vi "ReadConfigFile.vi"(8 "ErrorIn":errorcluster, 11 "ClusterIn":T1={"Admin"={"Lvl"=enum."Admin", "Pwd"=""}, "RTConfig"={"Arm"=FALSE, "Number"=0.0, "String"=""}, "SMS"={"Enbl?"=FALSE, "Addr"=[]}, "FPGA"={"Target"=enum."4", "Channel"=enum."4", "Ref1"=refnum, "Ref2"=refnum}, "Config"={"UsrCfg"={"Paths"={"CfgFile"=path "", "LogFolder"=path "", "LogFile"=path "", "NAS path"=path "", "ThreshFile"=path "", "RedunFolder"=path ""}, "SampleRate"=12500.0}, "FP_User"={"#NoiseSums"=1, "Max_df"=1, "AvgAvg"=FALSE, "#Avg"=1, "AutoCenter"=FALSE, "Inclin"={"Vmin"=0.0, "Vmax"=0.0, "Angle_min"=0.0, "Angle_max"=0.0, "Offset"=0.0, "Pos_Neg"=FALSE}, "1"={"Cal_"={"Fine"=0.999969482421875, "Coarse_"=10000.0}, "Beac"={"Fine"=4194303.0, "Coarse_"=1.0}, "Scale"={"Step4"=10000.0, "Step5"=4194303.0, "Step6"=1.0, "Step7"=10000.0}, "Offset"=1.0, "Scale_Noise"=12500.0, "Scale_Step1"=65535.0, "Scale_In_RT"=1.0, "ScaleMeas"=0.999969482421875, "FreqsToRemove"=[0, 1633], "Width"=[0, 1633], "ScaleMeasEnum"=enum."50", "FilterEnab"=enum."Step 1"}, "2"={"Cal_"={"Fine"=0.000213623046875, "Coarse_"=4194303.0}, "Beac"={"Fine"=0.000213623046875, "Coarse_"=4194303.0}, "Scale"={"Step4"=0.0, "Step5"=4194303.0, "Step6"=1.0, "Step7"=10000.0}, "Offset"=0.0, "Scale_Noise"=4194303.0, "Scale_Step1"=65535.0, "Scale_In_RT"=1.0, "ScaleMeas"=0.999969482421875, "FreqsToRemove"=[0, 1633], "Width"=[0, 1633], "ScaleMeasEnum"=enum."50", "FilterEnab"=enum."Step 1"}, "3"={"Cal_"={"Fine"=0.000213623046875, "Coarse_"=4194303.0}, "Beac"={"Fine"=0.000213623046875, "Coarse_"=4194303.0}, "Scale"={"Step4"=0.0, "Step5"=4194303.0, "Step6"=1.0, "Step7"=10000.0}, "Offset"=0.0, "Scale_Noise"=4194303.0, "Scale_Step1"=65535.0, "Scale_In_RT"=1.0, "ScaleMeas"=0.999969482421875, "FreqsToRemove"=[0, 1633], "Width"=[0, 1633], "ScaleMeasEnum"=enum."50", "FilterEnab"=enum."Step 1"}, "4"={"Cal_"={"Fine"=0.000213623046875, "Coarse_"=4194303.0}, "Beac"={"Fine"=0.000213623046875, "Coarse_"=4194303.0}, "Scale"={"Step4"=0.0, "Step5"=4194303.0, "Step6"=1.0, "Step7"=10000.0}, "Offset"=0.0, "Scale_Noise"=4194303.0, "Scale_Step1"=1.0, "Scale_In_RT"=10000.0, "ScaleMeas"=0.999969482421875, "FreqsToRemove"=[0, 1633], "Width"=[0, 1633], "ScaleMeasEnum"=enum."50", "FilterEnab"=enum."Step 1"}, "Target to Probe"=enum."4", "SNR_Thresh"=1.0, "Paths"={"CfgFile"=path "", "LogFolder"=path "", "LogFile"=path "", "NAS path"=path "", "ThreshFile"=path "", "RedunFolder"=path ""}, "Connex_Location"="", "SimulateFPGA"=FALSE, "Deadband"=0.0}}, "Stat"={"SysState"=enum."Init", "TrackRate"=FALSE, "AutoCentr"=FALSE}, "Alarm"={"TC13"={"Enbl"=FALSE, "ErrsAndWarns"={0.0, 5.663716814159292, 7.168141592920354, 8.584070796460177}}, "AI1"={"Enbl"=FALSE, "ErrsAndWarns"={0.0, 5.663716814159292, 7.168141592920354, 8.584070796460177}}, "AI2"={"Enbl"=FALSE, "ErrsAndWarns"={0.0, 5.663716814159292, 7.168141592920354, 8.584070796460177}}, "AI3"={"Enbl"=FALSE, "ErrsAndWarns"={0.0, 5.663716814159292, 7.168141592920354, 8.584070796460177}}, "AI4"={"Enbl"=FALSE, "ErrsAndWarns"={0.0, 5.663716814159292, 7.168141592920354, 8.584070796460177}}, "AI5"={"Enbl"=FALSE, "ErrsAndWarns"={0.0, 5.663716814159292, 7.168141592920354, 8.584070796460177}}, "AI6"={"Enbl"=FALSE, "ErrsAndWarns"={0.0, 5.663716814159292, 7.168141592920354, 8.584070796460177}}, "AI18"={"Enbl"=FALSE, "ErrsAndWarns"={0.0, 5.663716814159292, 7.168141592920354, 8.584070796460177}}, "AI19"={"Enbl"=FALSE, "ErrsAndWarns"={0.0, 5.663716814159292, 7.168141592920354, 8.584070796460177}}, "TE1"={"Enbl"=FALSE, "ErrsAndWarns"={0.0, 5.663716814159292, 7.168141592920354, 8.584070796460177}}, "TE2"={"Enbl"=TRUE, "ErrsAndWarns"={0.0, 5.663716814159292, 7.168141592920354, 8.584070796460177}}, "TE3"={"Enbl"=FALSE, "ErrsAndWarns"={0.0, 5.663716814159292, 7.168141592920354, 8.584070796460177}}, "ADAM1"={"Enbl"=FALSE, "ErrsAndWarns"={0.0, 5.663716814159292, 7.168141592920354, 8.584070796460177}}, "ADAM2"={"Enbl"=FALSE, "ErrsAndWarns"={0.0, 5.663716814159292, 7.168141592920354, 8.584070796460177}}, "ADAM3"={"Enbl"=FALSE, "ErrsAndWarns"={0.0, 5.663716814159292, 7.168141592920354, 8.584070796460177}}, "ADAM4"={"Enbl"=FALSE, "ErrsAndWarns"={0.0, 5.663716814159292, 7.168141592920354, 8.584070796460177}}, "72CoBeacFreq"={"Enbl"=FALSE, "ErrsAndWarns"={0.0, 5.663716814159292, 7.168141592920354, 8.584070796460177}}, "72CoCalFreq"={"Enbl"=FALSE, "ErrsAndWarns"={0.0, 5.663716814159292, 7.168141592920354, 8.584070796460177}}, "84CoBeacFreq"={"Enbl"=FALSE, "ErrsAndWarns"={0.0, 5.663716814159292, 7.168141592920354, 8.584070796460177}}, "84CoCalFreq"={"Enbl"=FALSE, "ErrsAndWarns"={0.0, 5.663716814159292, 7.168141592920354, 8.584070796460177}}, "72Co_CalTonePwr"={"Enbl"=FALSE, "ErrsAndWarns"={0.0, 5.663716814159292, 7.168141592920354, 8.584070796460177}}, "72X_CalTonePwr"={"Enbl"=FALSE, "ErrsAndWarns"={0.0, 5.663716814159292, 7.168141592920354, 8.584070796460177}}, "84Co_CalTonePwr"={"Enbl"=FALSE, "ErrsAndWarns"={0.0, 5.663716814159292, 7.168141592920354, 8.584070796460177}}, "84X_CalTonePwr"={"Enbl"=FALSE, "ErrsAndWarns"={0.0, 5.663716814159292, 7.168141592920354, 8.584070796460177}}}} {"Alarm"."84X_CalTonePwr"."ErrsAndWarns" scale=-120.0..-45.0; "Alarm"."72X_CalTonePwr"."ErrsAndWarns" scale=-120.0..-45.0; "Alarm"."84Co_CalTonePwr"."ErrsAndWarns" scale=-120.0..-45.0; "Alarm"."72Co_CalTonePwr"."ErrsAndWarns" scale=-120.0..-45.0; "Alarm"."84CoCalFreq"."ErrsAndWarns" scale=24.9..25.1; "Alarm"."84CoBeacFreq"."ErrsAndWarns" scale=25.5..27.0; "Alarm"."72CoCalFreq"."ErrsAndWarns" scale=24.9..25.1; "Alarm"."72CoBeacFreq"."ErrsAndWarns" scale=25.5..27.0; "Alarm"."ADAM4"."ErrsAndWarns" scale=30.0..52.0; "Alarm"."ADAM3"."ErrsAndWarns" scale=30.0..52.0; "Alarm"."ADAM2"."ErrsAndWarns" scale=30.0..52.0; "Alarm"."ADAM1"."ErrsAndWarns" scale=30.0..52.0; "Alarm"."TE3"."ErrsAndWarns" scale=30.0..52.0; "Alarm"."TE2"."ErrsAndWarns" scale=30.0..52.0; "Alarm"."TE1"."ErrsAndWarns" scale=20.0..52.0; "Alarm"."AI19"."ErrsAndWarns" scale=0.0..60.0; "Alarm"."AI18"."ErrsAndWarns" scale=-10.0..10.0; "Alarm"."AI6"."ErrsAndWarns" scale=0.0..35.0; "Alarm"."AI5"."ErrsAndWarns" scale=0.0..20.0; "Alarm"."AI4"."ErrsAndWarns" scale=0.0..15.0; "Alarm"."AI3"."ErrsAndWarns" scale=0.0..10.0; "Alarm"."AI2"."ErrsAndWarns" scale=0.0..10.0; "Alarm"."TC13"."ErrsAndWarns" scale=-10.0..40.0; "Config"."FP_User"."Deadband" format="%#.0f"}) -> (0 "ErrorOut":errorcluster, 2 "dup path":path, 3 "ClusterOut":T1={"Admin"={"Lvl"=enum."Admin", "Pwd"=""}, "RTConfig"={"Arm"=FALSE, "Number"=0.0, "String"=""}, "SMS"={"Enbl?"=FALSE, "Addr"=[]}, "FPGA"={"Target"=enum."4", "Channel"=enum."4", "Ref1"=refnum, "Ref2"=refnum}, "Config"={"UsrCfg"={"Paths"={"CfgFile"=path "", "LogFolder"=path "", "LogFile"=path "", "NAS path"=path "", "ThreshFile"=path "", "RedunFolder"=path ""}, "SampleRate"=12500.0}, "FP_User"={"#NoiseSums"=1, "Max_df"=1, "AvgAvg"=FALSE, "#Avg"=1, "AutoCenter"=FALSE, "Inclin"={"Vmin"=0.0, "Vmax"=0.0, "Angle_min"=0.0, "Angle_max"=0.0, "Offset"=0.0, "Pos_Neg"=FALSE}, "1"={"Cal_"={"Fine"=0.999969482421875, "Coarse_"=10000.0}, "Beac"={"Fine"=4194303.0, "Coarse_"=1.0}, "Scale"={"Step4"=10000.0, "Step5"=4194303.0, "Step6"=1.0, "Step7"=10000.0}, "Offset"=1.0, "Scale_Noise"=12500.0, "Scale_Step1"=65535.0, "Scale_In_RT"=1.0, "ScaleMeas"=0.999969482421875, "FreqsToRemove"=[0, 1633], "Width"=[0, 1633], "ScaleMeasEnum"=enum."50", "FilterEnab"=enum."Step 1"}, "2"={"Cal_"={"Fine"=0.000213623046875, "Coarse_"=4194303.0}, "Beac"={"Fine"=0.000213623046875, "Coarse_"=4194303.0}, "Scale"={"Step4"=0.0, "Step5"=4194303.0, "Step6"=1.0, "Step7"=10000.0}, "Offset"=0.0, "Scale_Noise"=4194303.0, "Scale_Step1"=65535.0, "Scale_In_RT"=1.0, "ScaleMeas"=0.999969482421875, "FreqsToRemove"=[0, 1633], "Width"=[0, 1633], "ScaleMeasEnum"=enum."50", "FilterEnab"=enum."Step 1"}, "3"={"Cal_"={"Fine"=0.000213623046875, "Coarse_"=4194303.0}, "Beac"={"Fine"=0.000213623046875, "Coarse_"=4194303.0}, "Scale"={"Step4"=0.0, "Step5"=4194303.0, "Step6"=1.0, "Step7"=10000.0}, "Offset"=0.0, "Scale_Noise"=4194303.0, "Scale_Step1"=65535.0, "Scale_In_RT"=1.0, "ScaleMeas"=0.999969482421875, "FreqsToRemove"=[0, 1633], "Width"=[0, 1633], "ScaleMeasEnum"=enum."50", "FilterEnab"=enum."Step 1"}, "4"={"Cal_"={"Fine"=0.000213623046875, "Coarse_"=4194303.0}, "Beac"={"Fine"=0.000213623046875, "Coarse_"=4194303.0}, "Scale"={"Step4"=0.0, "Step5"=4194303.0, "Step6"=1.0, "Step7"=10000.0}, "Offset"=0.0, "Scale_Noise"=4194303.0, "Scale_Step1"=1.0, "Scale_In_RT"=10000.0, "ScaleMeas"=0.999969482421875, "FreqsToRemove"=[0, 1633], "Width"=[0, 1633], "ScaleMeasEnum"=enum."50", "FilterEnab"=enum."Step 1"}, "Target to Probe"=enum."4", "SNR_Thresh"=1.0, "Paths"={"CfgFile"=path "", "LogFolder"=path "", "LogFile"=path "", "NAS path"=path "", "ThreshFile"=path "", "RedunFolder"=path ""}, "Connex_Location"="", "SimulateFPGA"=FALSE, "Deadband"=0.0}}, "Stat"={"SysState"=enum."Init", "TrackRate"=FALSE, "AutoCentr"=FALSE}, "Alarm"={"TC13"={"Enbl"=FALSE, "ErrsAndWarns"={0.0, 5.663716814159292, 7.168141592920354, 8.584070796460177}}, "AI1"={"Enbl"=FALSE, "ErrsAndWarns"={0.0, 5.663716814159292, 7.168141592920354, 8.584070796460177}}, "AI2"={"Enbl"=FALSE, "ErrsAndWarns"={0.0, 5.663716814159292, 7.168141592920354, 8.584070796460177}}, "AI3"={"Enbl"=FALSE, "ErrsAndWarns"={0.0, 5.663716814159292, 7.168141592920354, 8.584070796460177}}, "AI4"={"Enbl"=FALSE, "ErrsAndWarns"={0.0, 5.663716814159292, 7.168141592920354, 8.584070796460177}}, "AI5"={"Enbl"=FALSE, "ErrsAndWarns"={0.0, 5.663716814159292, 7.168141592920354, 8.584070796460177}}, "AI6"={"Enbl"=FALSE, "ErrsAndWarns"={0.0, 5.663716814159292, 7.168141592920354, 8.584070796460177}}, "AI18"={"Enbl"=FALSE, "ErrsAndWarns"={0.0, 5.663716814159292, 7.168141592920354, 8.584070796460177}}, "AI19"={"Enbl"=FALSE, "ErrsAndWarns"={0.0, 5.663716814159292, 7.168141592920354, 8.584070796460177}}, "TE1"={"Enbl"=FALSE, "ErrsAndWarns"={0.0, 5.663716814159292, 7.168141592920354, 8.584070796460177}}, "TE2"={"Enbl"=TRUE, "ErrsAndWarns"={0.0, 5.663716814159292, 7.168141592920354, 8.584070796460177}}, "TE3"={"Enbl"=FALSE, "ErrsAndWarns"={0.0, 5.663716814159292, 7.168141592920354, 8.584070796460177}}, "ADAM1"={"Enbl"=FALSE, "ErrsAndWarns"={0.0, 5.663716814159292, 7.168141592920354, 8.584070796460177}}, "ADAM2"={"Enbl"=FALSE, "ErrsAndWarns"={0.0, 5.663716814159292, 7.168141592920354, 8.584070796460177}}, "ADAM3"={"Enbl"=FALSE, "ErrsAndWarns"={0.0, 5.663716814159292, 7.168141592920354, 8.584070796460177}}, "ADAM4"={"Enbl"=FALSE, "ErrsAndWarns"={0.0, 5.663716814159292, 7.168141592920354, 8.584070796460177}}, "72CoBeacFreq"={"Enbl"=FALSE, "ErrsAndWarns"={0.0, 5.663716814159292, 7.168141592920354, 8.584070796460177}}, "72CoCalFreq"={"Enbl"=FALSE, "ErrsAndWarns"={0.0, 5.663716814159292, 7.168141592920354, 8.584070796460177}}, "84CoBeacFreq"={"Enbl"=FALSE, "ErrsAndWarns"={0.0, 5.663716814159292, 7.168141592920354, 8.584070796460177}}, "84CoCalFreq"={"Enbl"=FALSE, "ErrsAndWarns"={0.0, 5.663716814159292, 7.168141592920354, 8.584070796460177}}, "72Co_CalTonePwr"={"Enbl"=FALSE, "ErrsAndWarns"={0.0, 5.663716814159292, 7.168141592920354, 8.584070796460177}}, "72X_CalTonePwr"={"Enbl"=FALSE, "ErrsAndWarns"={0.0, 5.663716814159292, 7.168141592920354, 8.584070796460177}}, "84Co_CalTonePwr"={"Enbl"=FALSE, "ErrsAndWarns"={0.0, 5.663716814159292, 7.168141592920354, 8.584070796460177}}, "84X_CalTonePwr"={"Enbl"=FALSE, "ErrsAndWarns"={0.0, 5.663716814159292, 7.168141592920354, 8.584070796460177}}}} {"Alarm"."84X_CalTonePwr"."ErrsAndWarns" scale=-120.0..-45.0; "Alarm"."72X_CalTonePwr"."ErrsAndWarns" scale=-120.0..-45.0; "Alarm"."84Co_CalTonePwr"."ErrsAndWarns" scale=-120.0..-45.0; "Alarm"."72Co_CalTonePwr"."ErrsAndWarns" scale=-120.0..-45.0; "Alarm"."84CoCalFreq"."ErrsAndWarns" scale=24.9..25.1; "Alarm"."84CoBeacFreq"."ErrsAndWarns" scale=25.5..27.0; "Alarm"."72CoCalFreq"."ErrsAndWarns" scale=24.9..25.1; "Alarm"."72CoBeacFreq"."ErrsAndWarns" scale=25.5..27.0; "Alarm"."ADAM4"."ErrsAndWarns" scale=30.0..52.0; "Alarm"."ADAM3"."ErrsAndWarns" scale=30.0..52.0; "Alarm"."ADAM2"."ErrsAndWarns" scale=30.0..52.0; "Alarm"."ADAM1"."ErrsAndWarns" scale=30.0..52.0; "Alarm"."TE3"."ErrsAndWarns" scale=30.0..52.0; "Alarm"."TE2"."ErrsAndWarns" scale=30.0..52.0; "Alarm"."TE1"."ErrsAndWarns" scale=20.0..52.0; "Alarm"."AI19"."ErrsAndWarns" scale=0.0..60.0; "Alarm"."AI18"."ErrsAndWarns" scale=-10.0..10.0; "Alarm"."AI6"."ErrsAndWarns" scale=0.0..35.0; "Alarm"."AI5"."ErrsAndWarns" scale=0.0..20.0; "Alarm"."AI4"."ErrsAndWarns" scale=0.0..15.0; "Alarm"."AI3"."ErrsAndWarns" scale=0.0..10.0; "Alarm"."AI2"."ErrsAndWarns" scale=0.0..10.0; "Alarm"."TC13"."ErrsAndWarns" scale=-10.0..40.0; "Config"."FP_User"."Deadband" format="%#.0f"})   [LabVIEW 2018]
doc: "Attempt to read the configuration (INI) file specified in ClusterIn.Paths.CfgFile. If the file exists, the INI file is read and elements are filled in to the cluster. If it does not exist, a new INI file is created using default values.\n\nAdd elements to this VI for each cluster element that you wish to reload.\n\nCopyright © 2019 Epimedia, Inc. All Rights Reserved.\n\nThe Epimedia Application Library is Copyright © 2009-2017 Epimedia, Inc. \nAll Rights Reserved. Used under license."
uses:
  Controls/MasterCluster.ctl
  Controls/Clusts/AdminCluster.ctl
  Controls/UserLevelEnum.ctl
  Controls/RT_Config.ctl
  Controls/SMSDataCluster.ctl
  Controls/Clusts/FPGA_Config_Clust.ctl
  Controls/Enums/TargetNumber.ctl
  Controls/Clusts/Config_Clust.ctl
  Controls/Clusts/UserConfig.ctl
  Controls/PathsCluster.ctl
  Controls/Clusts/FrontPanel_UserConfig.ctl
  Controls/Clusts/Inclinometer_User_Cfg.ctl
  Controls/Clusts/FP_UserTargetConfig.ctl
  Controls/Clusts/FreqShift.ctl
  Controls/Clusts/FPGA_Scale.ctl
  Controls/Enums/ScaleMeasure.ctl
  Controls/RadioButtons/FilterEnableRadio.ctl
  Controls/SystemStatusCluster.ctl
  Controls/SystemStateEnum.ctl
  Controls/Clusts/AlarmSettingsClust.ctl
  Controls/Clusts/AlarmThresh_OneChan.ctl
  <vilib>/Utility/sysdir.llb/System Directory Type.ctl
  <vilib>/Utility/xml.llb/Read From XML File(string).vi
  <vilib>/Utility/config.llb/NI_LVConfig.lvlib
  <vilib>/Utility/config.llb/Read Key (Path).vi
  <vilib>/Utility/config.llb/Read Key (String).vi
panel:
  # "Copyright © 2019 Epimedia, Inc. All Rights Reserved.\n\nThe Epimedia Application Library is Copyright © 2009-2017 Epimedia, Inc. \nAll Rights Reserved. Used under license."
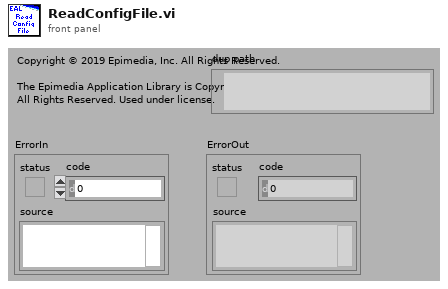
[diagram p1: front panel]
types:
  T1 = typedef "MasterCluster.ctl" = cluster{"Admin":T2, "RTConfig":T4, "SMS":T5, "FPGA":T6, "Config":T8, "Stat":T18, "Alarm":T20}
  T2 = typedef "AdminCluster.ctl" = cluster{"Lvl":T3, "Pwd":string}
  T3 = typedef "UserLevelEnum.ctl" = enum16{"Admin", "Operator"}
  T4 = typedef "RT_Config.ctl" = cluster{"Arm":bool, "Number":dbl, "String":string}
  T5 = typedef "SMSDataCluster.ctl" = cluster{"Enbl?":bool, "Addr":string[]}
  T6 = typedef "FPGA_Config_Clust.ctl" = cluster{"Target":T7, "Channel":T7, "Ref1":refnum<k20>, "Ref2":refnum<k20>}
  T7 = typedef "TargetNumber.ctl" = enum16{"1", "2", "3", "4"}
  T8 = typedef "Config_Clust.ctl" = cluster{"UsrCfg":T9, "FP_User":T11}
  T9 = typedef "UserConfig.ctl" = cluster{"Paths":T10, "SampleRate":dbl}
  T10 = typedef "PathsCluster.ctl" = cluster{"CfgFile":path, "LogFolder":path, "LogFile":path, "NAS path":path, "ThreshFile":path, "RedunFolder":path}
  T11 = typedef "FrontPanel_UserConfig.ctl" = cluster{"#NoiseSums":u32, "Max_df":u32, "AvgAvg":bool, "#Avg":u16, "AutoCenter":bool, "Inclin":T12, "1":T13, "2":T13, "3":T13, "4":T13, "Target to Probe":T7, "SNR_Thresh":dbl, "Paths":T10, "Connex_Location":string, "SimulateFPGA":bool, "Deadband":dbl}
  T12 = typedef "Inclinometer_User_Cfg.ctl" = cluster{"Vmin":dbl, "Vmax":dbl, "Angle_min":dbl, "Angle_max":dbl, "Offset":dbl, "Pos_Neg":bool}
  T13 = typedef "FP_UserTargetConfig.ctl" = cluster{"Cal_":T14, "Beac":T14, "Scale":T15, "Offset":fxp<+/-,16,16>, "Scale_Noise":fxp<+/-,30,30>, "Scale_Step1":fxp<+/-,17,17>, "Scale_In_RT":ext, "ScaleMeas":fxp<+/-,16,1>, "FreqsToRemove":i32[], "Width":i32[], "ScaleMeasEnum":T16, "FilterEnab":T17}
  T14 = typedef "FreqShift.ctl" = cluster{"Fine":dbl, "Coarse_":dbl}
  T15 = typedef "FPGA_Scale.ctl" = cluster{"Step4":fxp<+/-,23,23>, "Step5":fxp<+/-,23,23>, "Step6":fxp<+/-,23,23>, "Step7":fxp<+/-,23,23>}
  T16 = typedef "ScaleMeasure.ctl" = enum16{"1", "10", "50", "42"}
  T17 = typedef "FilterEnableRadio.ctl" = enum32{"None", "Step 1", "Frequency Shift", "Step 4", "Step 5", "Step 6", "Step 7"}
  T18 = typedef "SystemStatusCluster.ctl" = cluster{"SysState":T19, "TrackRate":bool, "AutoCentr":bool}
  T19 = typedef "SystemStateEnum.ctl" = enum16{"Init", "Idle", "Running", "System Fault", "System Error", "Exit"}
  T20 = typedef "AlarmSettingsClust.ctl" = cluster{"TC13":T21, "AI1":T21, "AI2":T21, "AI3":T21, "AI4":T21, "AI5":T21, "AI6":T21, "AI18":T21, "AI19":T21, "TE1":T21, "TE2":T21, "TE3":T21, "ADAM1":T21, "ADAM2":T21, "ADAM3":T21, "ADAM4":T21, "72CoBeacFreq":T21, "72CoCalFreq":T21, "84CoBeacFreq":T21, "84CoCalFreq":T21, "72Co_CalTonePwr":T21, "72X_CalTonePwr":T21, "84Co_CalTonePwr":T21, "84X_CalTonePwr":T21}
  T21 = typedef "AlarmThresh_OneChan.ctl" = cluster{"Enbl":bool, "ErrsAndWarns":cluster{dbl, dbl, dbl, dbl}}
  T22 = typedef "System Directory Type.ctl" = i32
  T23 = typedef "NI_LVConfig.lvlib/Config Data RefNum.ctl" = refnum<k1>
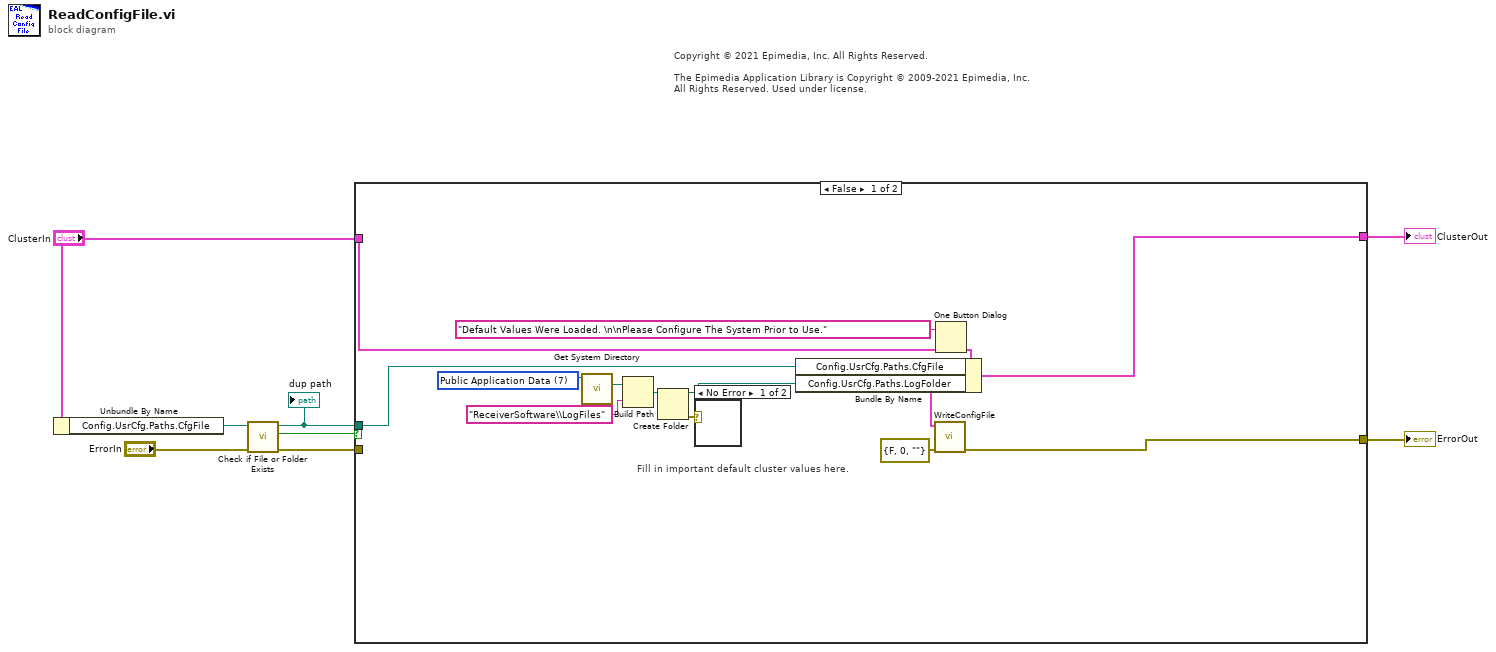
[diagram p0: block diagram]
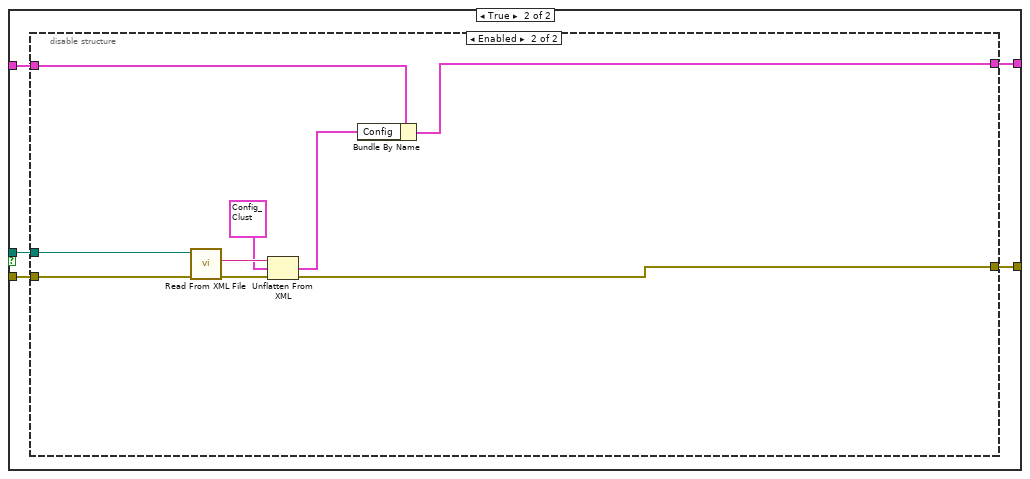
[diagram p3: hidden frame]
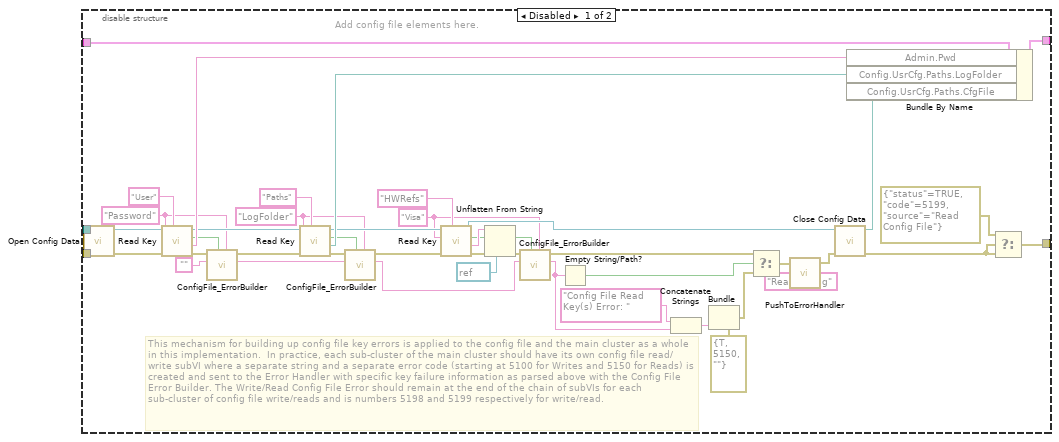
[diagram p4: hidden frame]
diagram:
  # "Copyright © 2021 Epimedia, Inc. All Rights Reserved.\n\nThe Epimedia Application Library is Copyright © 2009-2021 Epimedia, Inc. \nAll Rights Reserved. Used under license."
  n1 = Unbundle By Name("ClusterIn") -> ("Config.UsrCfg.Paths.CfgFile"=w5:path)
  n2 = call <vilib>:"Check if File or Folder Exists.vi"("error in (no error)"="ErrorIn", "path"=w5) -> ("error out"=w1:errorcluster, "file or folder exists?"=w2:bool, "dup path"=w4:path)  [unwired: 7 out]
  "dup path" <- w4
  n3 = case shown="False" w2 {
    tunnel: [w20 w21] -> w8
    tunnel: [w18 w25] -> w7
    tunnel: w4 -> [w15 w24]
    tunnel: "ClusterIn" -> [w17 w23]
    tunnel: w1 -> [_ w22]
    frame False {
      w14 = T22 7 items=["User Home"=0, "User Desktop"=1, "User Documents"=2, "User Application Data"=3, "User Preferences"=4, "User Temporary"=5, "Public Documents"=6, "Public Application Data"=7, "Public Preferences"=8, "Public Cache"=13, "System Core Libraries"=9, "System Installed Libraries"=10, "Application Files"=11, "Boot Volume Root"=12] ("system directory type")
      # "Fill in important default cluster values here."
      n4 = call <vilib>:"Get System Directory.vi"("system directory type"=w14) -> ("system directory"=w11:path)  [unwired: 10 in]
      n5 = Build Path(base path=w11, name or relative path="ReceiverSoftware\\LogFiles") -> (appended path=w10:path)
      n6 = Create Folder(path (use dialog)=w10) -> (created path=w9:path, error out=w12:errorcluster)  [unwired: 2 in, 1 out]
      n7 = case shown="No Error" w12 {
        frame No Error {
        }
        frame Error {
        }
      }
      n8 = Bundle By Name(cluster=w17, "Config.UsrCfg.Paths.CfgFile"=w15, "Config.UsrCfg.Paths.LogFolder"=w9) -> (w18:T1)
      n9 = call "WriteConfigFile.vi"("ErrorIn"=errorcluster {"status"=FALSE, "code"=0, "source"=""}, "ClusterIn"=w18) -> ("ErrorOut"=w20:errorcluster)  [unwired: 1 in, 8 out]
      n10 = One Button Dialog(message="Default Values Were Loaded. \n\nPlease Configure The System Prior to Use.") -> ()  [unwired: 2 out]
    }
    frame True {
      n11 = disable-structure shown="Enabled" {
        disable-tunnel: [w69 w73] -> w25
        disable-tunnel: w24 -> [w66 w78]
        disable-tunnel: w23 -> [w65 w74]
        disable-tunnel: w22 -> [w64 w79]
        disable-tunnel: [w26 w76] -> w21
        frame Disabled {
          w50 = "Password" ("key")
          w40 = "Visa" ("key")
          w45 = "LogFolder" ("key")
          # "This mechanism for building up config file key errors is applied to the config file and the main cluster as a whole in this implementation.  In practice, each sub-cluster of the main cluster should have its own config file read/write subVI where a separate string and a separate error code (starting at 5100 for Writes and 5150 for Reads) is created and sent to the Error Handler with specific key failure information as parsed above with the Config File Error Builder. The Write/Read Config File Error should remain at the end of the chain of subVIs for each sub-cluster of config file write/reads and is numbers 5198 and 5199 respectively for write/read."
          # "Add config file elements here."
          n12 = call <vilib>:"Open Config Data.vi"("error in (no error)"=w64, "configuration file path"=w66) -> ("error out"=w60:errorcluster, "refnum"=w59:T23)  [unwired: 7 in, 1 out]
          n13 = call-poly <vilib>:"Read Key.vi"("section"="User" ("key"), "error in (no error)"=w60, "key"=w50, "refnum"=w59) -> ("error out"=w52:errorcluster, "value"=w63:string, "found?"=w49:bool, "refnum out"=w54:T23)  [unwired: 2 in, 2 out]
          n14 = call "ConfigFile_ErrorBuilder.vi"("KeyNameIn"=w50, "KeyFound?"=w49, "IncomingErrorString"="", "ErrorIn"=w52) -> ("OutgoingErrorString"=w43:string, "ErrorOut"=w51:errorcluster)  [unwired: 6 in]
          n15 = call-poly <vilib>:"Read Key.vi"("section"="Paths" ("key"), "error in (no error)"=w51, "key"=w45, "refnum"=w54) -> ("error out"=w46:errorcluster, "value"=w56:path, "found?"=w44:bool, "refnum out"=w53:T23)  [unwired: 1 in, 3 out]
          n16 = call "ConfigFile_ErrorBuilder.vi"("KeyNameIn"=w45, "KeyFound?"=w44, "IncomingErrorString"=w43, "ErrorIn"=w46) -> ("OutgoingErrorString"=w41:string, "ErrorOut"=w42:errorcluster)  [unwired: 6 in]
          n17 = call-poly <vilib>:"Read Key.vi"("section"="HWRefs" ("key"), "error in (no error)"=w42, "key"=w40, "refnum"=w53) -> ("error out"=w68:errorcluster, "value"=w67:string, "found?"=w39:bool, "refnum out"=w55:T23)  [unwired: 2 in, 2 out]
          n18 = Unflatten From String(type=refnum<visa-resource-name> refnum ("Refs.SRSVisa"), binary string=w67, error in (no error)=w68) -> (error out=w47:errorcluster)  [unwired: 4 out]
          n19 = call "ConfigFile_ErrorBuilder.vi"("KeyNameIn"=w40, "KeyFound?"=w39, "IncomingErrorString"=w41, "ErrorIn"=w47) -> ("OutgoingErrorString"=w34:string, "ErrorOut"=w32:errorcluster)  [unwired: 6 in]
          n20 = Empty String/Path?(string/path=w34) -> (empty?=w33:bool)
          n21 = Concatenate Strings("Config File Read Key(s) Error: " ("source"), w34) -> (w35:string)
          n22 = Bundle(cluster=errorcluster {"status"=TRUE, "code"=5150, "source"=""} ("ErrorIn"), "source"=w35) -> (w38:errorcluster)  [unwired: 2 in]
          n23 = Select(t=w32, s=w33, f=w38) -> (s? t:f=w30:errorcluster)
          n24 = call "PushToErrorHandler.vi"("ErrorIn"=w30, "ErrorLocation"="Read Config") -> ("ErrorOut"=w29:errorcluster)  [unwired: 5 in]
          n25 = call <vilib>:"Close Config Data.vi"("error in (no error)"=w29, "refnum"=w55) -> ("error out"=w27:errorcluster, "file path"=w70:path)  [unwired: 1 in, 7 out]
          n26 = Bundle By Name(cluster=w65, "Admin.Pwd"=w63, "Config.UsrCfg.Paths.LogFolder"=w56, "Config.UsrCfg.Paths.CfgFile"=w70) -> (w69:T1)
          n27 = Select(t=errorcluster {"status"=TRUE, "code"=5199, "source"="Read Config File"} ("f"), s=w27, f=w27) -> (s? t:f=w26:errorcluster)
        }
        frame Enabled {
          n28 = call-poly <vilib>:"Read From XML File.vi"("error in (no error)"=w79, "XML File Path"=w78) -> ("error out"=w77:errorcluster, "XML Elements"=w75:string)  [unwired: 7 in, 1 out]
          n29 = Unflatten From XML(xml string=w75, type=T8 {"UsrCfg"={"Paths"={"CfgFile"=path "", "LogFolder"=path "", "LogFile"=path "", "NAS path"=path "", "ThreshFile"=path "", "RedunFolder"=path ""}, "SampleRate"=12500.0}, "FP_User"={"#NoiseSums"=1, "Max_df"=1, "AvgAvg"=FALSE, "#Avg"=1, "AutoCenter"=FALSE, "Inclin"={"Vmin"=0.0, "Vmax"=0.0, "Angle_min"=0.0, "Angle_max"=0.0, "Offset"=0.0, "Pos_Neg"=FALSE}, "1"={"Cal_"={"Fine"=0.000213623046875, "Coarse_"=4194303.0}, "Beac"={"Fine"=4194303.0, "Coarse_"=1.0}, "Scale"={"Step4"=10000.0, "Step5"=4194303.0, "Step6"=1.0, "Step7"=10000.0}, "Offset"=0.0, "Scale_Noise"=4194303.0, "Scale_Step1"=65535.0, "Scale_In_RT"=1.0, "ScaleMeas"=0.999969482421875, "FreqsToRemove"=[0, 1633], "Width"=[0, 1633], "ScaleMeasEnum"=enum."50", "FilterEnab"=enum."Step 1"}, "2"={"Cal_"={"Fine"=0.000213623046875, "Coarse_"=4194303.0}, "Beac"={"Fine"=0.000213623046875, "Coarse_"=4194303.0}, "Scale"={"Step4"=0.0, "Step5"=4194303.0, "Step6"=1.0, "Step7"=10000.0}, "Offset"=0.0, "Scale_Noise"=4194303.0, "Scale_Step1"=65535.0, "Scale_In_RT"=1.0, "ScaleMeas"=0.999969482421875, "FreqsToRemove"=[0, 1633], "Width"=[0, 1633], "ScaleMeasEnum"=enum."50", "FilterEnab"=enum."Step 1"}, "3"={"Cal_"={"Fine"=0.000213623046875, "Coarse_"=4194303.0}, "Beac"={"Fine"=0.000213623046875, "Coarse_"=4194303.0}, "Scale"={"Step4"=0.0, "Step5"=4194303.0, "Step6"=1.0, "Step7"=10000.0}, "Offset"=0.0, "Scale_Noise"=4194303.0, "Scale_Step1"=65535.0, "Scale_In_RT"=1.0, "ScaleMeas"=0.999969482421875, "FreqsToRemove"=[0, 1633], "Width"=[0, 1633], "ScaleMeasEnum"=enum."50", "FilterEnab"=enum."Step 1"}, "4"={"Cal_"={"Fine"=0.000213623046875, "Coarse_"=4194303.0}, "Beac"={"Fine"=0.000213623046875, "Coarse_"=4194303.0}, "Scale"={"Step4"=0.0, "Step5"=4194303.0, "Step6"=1.0, "Step7"=10000.0}, "Offset"=0.0, "Scale_Noise"=4194303.0, "Scale_Step1"=1.0, "Scale_In_RT"=10000.0, "ScaleMeas"=0.999969482421875, "FreqsToRemove"=[0, 1633], "Width"=[0, 1633], "ScaleMeasEnum"=enum."50", "FilterEnab"=enum."Step 1"}, "Target to Probe"=enum."4", "SNR_Thresh"=1.0, "Paths"={"CfgFile"=path "", "LogFolder"=path "", "LogFile"=path "", "NAS path"=path "", "ThreshFile"=path "", "RedunFolder"=path ""}, "Connex_Location"="", "SimulateFPGA"=FALSE, "Deadband"=0.0}} ("Config"), error in (no error)=w77) -> (value=w72:T8, error out=w76:errorcluster)
          n30 = Bundle By Name(cluster=w74, "Config"=w72) -> (w73:T1)
        }
      }
    }
  }
  "ErrorOut" <- w8
  "ClusterOut" <- w7
